vi "Get Tree Items.vi"(8 "error in (no error)":errorcluster, 10 "Filter":T1, 11 "Result Model by Reference In":refnum<class "Result Model by Reference.lvclass">) -> (0 "error out":errorcluster, 2 "Tree Items":T2(array[cluster]))   [LabVIEW 2020, in "Result Model by Reference.lvclass"]
uses:
  Result Model by Reference.lvclass
  Result Model by Reference.lvclass/Result Model by Reference.ctl
  Result Model/Result Model.lvclass
  Result Model/Tree Item Filter.ctl
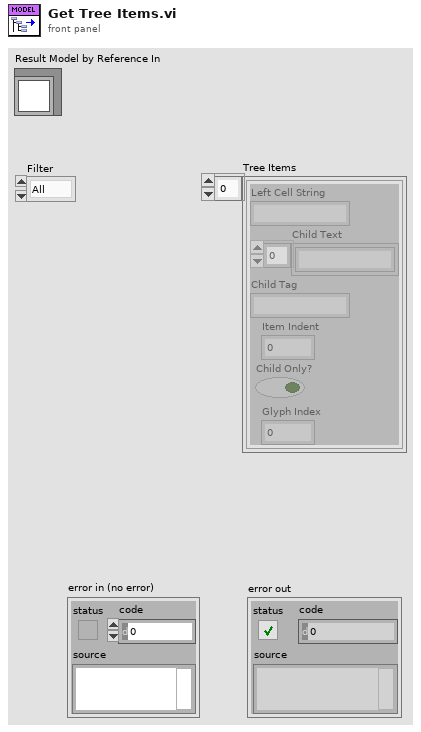
[diagram p1: front panel]
types:
  T1 = typedef "Result Model.lvclass/Tree Item Filter.ctl" = enum16{"All", "Only Fails", "Fails or else Not Executed"}
  T2 = cluster{"Left Cell String":string, "Child Text":string[], "Child Tag":string, "Item Indent":i32, "Child Only?":bool, "Glyph Index":i32}[]
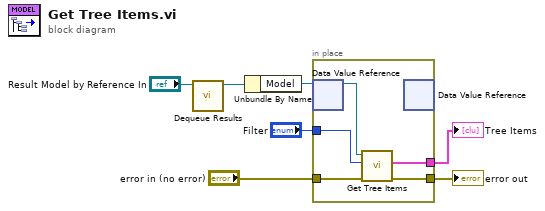
[diagram p0: block diagram]
diagram:
  n1 = call "Dequeue Results.vi"("Result Model by Reference in"="Result Model by Reference In") -> ("Result Model by Reference out"=w1:refnum<class "Result Model by Reference.lvclass">)  [unwired: 10 in]
  n2 = Unbundle By Name(w1) -> ("Model"=w7:refnum<data-value>)
  n3 = in-place {
    in-place-border: "error in (no error)" -> [w12]
    in-place-border: [w11] -> w3
    in-place-border: "Filter" -> [w9]
    in-place-border: [w8] -> w2
    n4 = in-place-dvr #1(w7) -> (w10:refnum<class "Result Model.lvclass">)  [unwired: 1 out]
    n5 = call "Get Tree Items.vi"("error in (no error)"=w12, "Filter"=w9, "Result Model In"=w10) -> ("error out"=w11:errorcluster, "Tree Items"=w8:T2)  [unwired: 7 in]
    n6 = in-place-dvr #1() -> ()  [unwired: 1 in, 2 out]
  }
  "Tree Items" <- w2
  "error out" <- w3
